vi "F206_Choose_SPI.vi"(1 "SPI in":cluster{"R":dbl, "S":dbl, "T":dbl}={"R"=-72.58, "S"=0.0, "T"=23.48} {"T" format="%.3f"; "S" format="%.3f"; "R" format="%.3f"}, 2 "SPI 1":bool caption="Boolean", 3 "SPI 2":bool caption="Boolean", 4 "SPI 3":bool caption="Boolean") -> (15 "SPI out":cluster{"R":dbl, "S":dbl, "T":dbl} {"T" format="%.3f"; "S" format="%.3f"; "R" format="%.3f"}, 16 "SPI 1 out":bool caption="Boolean", 17 "SPI 2 out":bool caption="Boolean", 18 "SPI 3 out":bool caption="Boolean")   [LabVIEW 2020]
doc: "F-206-specific. Returns coordinates for Pivot Point depending on states of buttons on schematic platform."
panel:
  # "F-206-specific. Returns coordinates for Pivot Point depending\non states of buttons on schematic platform."
  # "Pivot Point Location in"
  # "Pivot Point Location out"
  # "mm"
  # "mm"
  # "mm"
  # "mm"
  # "mm"
  # "mm"
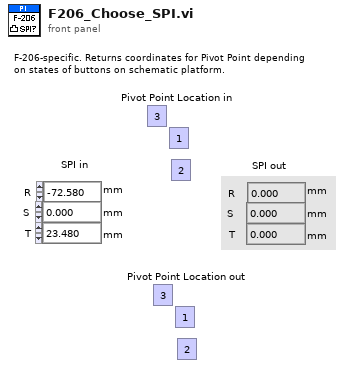
[diagram p1: front panel]
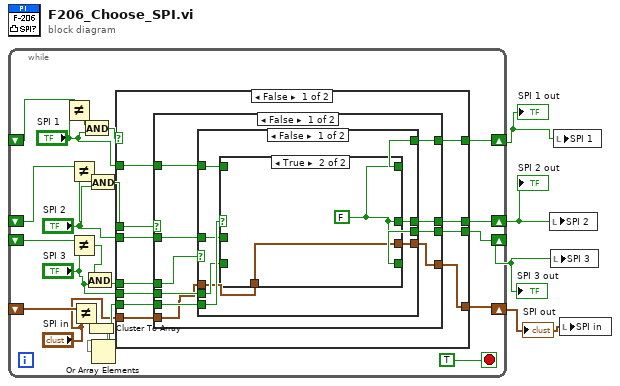
[diagram p0: block diagram]
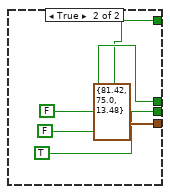
[diagram p3: hidden frame]
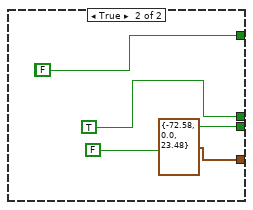
[diagram p4: hidden frame]
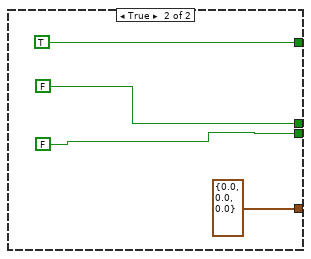
[diagram p5: hidden frame]
diagram:
  n1 = while {
    shift-right: [w25] -> w3
    shift-left: _ -> [w26]
    shift-right: [w24] -> w4
    shift-left: _ -> [w22]
    shift-right: [w23] -> w2
    shift-left: _ -> [w21]
    shift-right: [w5] -> w1
    shift-left: _ -> [w10]
    stop <- TRUE stop-if-true
    n2 = Not Equal?(x=w26, y="SPI 1") -> (x != y?=w19:bool)
    n3 = Not Equal?(x=w22, y="SPI 2") -> (x != y?=w17:bool)
    n4 = Not Equal?(x=w21, y="SPI 3") -> (x != y?=w15:bool)
    n5 = Not Equal?(x=w10, y="SPI in") -> (x != y?=w9:cluster{"R":bool, "S":bool, "T":bool})
    n6 = And(x=w19, y="SPI 1") -> (x .and. y?=w18:bool)
    n7 = And(x=w15, y="SPI 3") -> (x .and. y?=w14:bool)
    n8 = Cluster To Array(cluster=w9) -> (array=w8:bool[])
    n9 = And(x=w17, y="SPI 2") -> (x .and. y?=w16:bool)
    n10 = Or Array Elements(Boolean array=w8) -> (logical OR=w7:bool)
    n11 = case shown="False" w18 {
      tunnel: [w37 cluster{"R":dbl, "S":dbl, "T":dbl} {"R"=0.0, "S"=0.0, "T"=0.0} ("SPI")] -> w5
      tunnel: [w35 TRUE] -> w25
      tunnel: w16 -> [w36 _]
      tunnel: [w34 FALSE] -> w24
      tunnel: [w33 FALSE] -> w23
      tunnel: w14 -> [w32 _]
      tunnel: "SPI 1" -> [w31 _]
      tunnel: "SPI 2" -> [w30 _]
      tunnel: "SPI 3" -> [w29 _]
      tunnel: w7 -> [w28 _]
      tunnel: "SPI in" -> [w27 _]
      frame False {
        n12 = case shown="False" w36 {
          tunnel: [w47 cluster{"R":dbl, "S":dbl, "T":dbl} {"R"=-72.58, "S"=0.0, "T"=23.48} ("SPI")] -> w37
          tunnel: [w44 FALSE] -> w35
          tunnel: [w46 TRUE] -> w34
          tunnel: [w45 FALSE] -> w33
          tunnel: w32 -> [w43 _]
          tunnel: w31 -> [w42 _]
          tunnel: w30 -> [w41 _]
          tunnel: w29 -> [w40 _]
          tunnel: w28 -> [w39 _]
          tunnel: w27 -> [w38 _]
          frame False {
            n13 = case shown="False" w43 {
              tunnel: [w48 cluster{"R":dbl, "S":dbl, "T":dbl} {"R"=81.42, "S"=75.0, "T"=13.48} ("SPI")] -> w47
              tunnel: [w52 FALSE] -> w46
              tunnel: [w50 TRUE] -> w45
              tunnel: [w55 FALSE] -> w44
              tunnel: w42 -> [w56 _]
              tunnel: w41 -> [w53 _]
              tunnel: w40 -> [w51 _]
              tunnel: w39 -> [w54 _]
              tunnel: w38 -> [w49 _]
              frame False {
                n14 = case shown="True" w54 {
                  tunnel: w56 -> [w60 _]
                  tunnel: [w60 w61] -> w55
                  tunnel: w53 -> [w59 _]
                  tunnel: [w59 w61] -> w52
                  tunnel: w51 -> [w58 _]
                  tunnel: [w58 w61] -> w50
                  tunnel: w49 -> [w57 w62]
                  tunnel: [w57 w62] -> w48
                  frame False {
                  }
                  frame True {
                    w61 = FALSE
                  }
                }
              }
              frame True {
              }
            }
          }
          frame True {
            (unwired) FALSE
          }
        }
      }
      frame True {
      }
    }
  }
  "SPI 2 out" <- w4
  "SPI 1 out" <- w3
  "SPI 3 out" <- w2
  "SPI out" <- w1
  n15 = local write "SPI 2"(w4) -> ()
  n16 = local write "SPI 3"(w2) -> ()
  n17 = local write "SPI 1"(w3) -> ()
  n18 = local write "SPI in"(w1) -> ()
